vi "Create Data Folder.vi"(8 "error in (no error)":errorcluster, 9 "Description":string, 10 "Name":string, 11 "Parent Section":refnum<k24>) -> (0 "error out":errorcluster, 2 "New Section":refnum<k24>, 3 "Parent Section Duplicate":refnum<k24>, 4 "Newly Created?":bool)   [LabVIEW 2010, in "RefMem PtByPt System Definition API.lvlib"]
doc: "Creates a new folder for orginizational purposes."
uses:
  RefMem PtByPt System Definition API.lvlib
  NationalInstruments.VeriStand.SystemDefinitionAPI
  Custom Device/Controls/Global.vi
  Custom Device/RefMem PtByPt Custom Device.lvlib
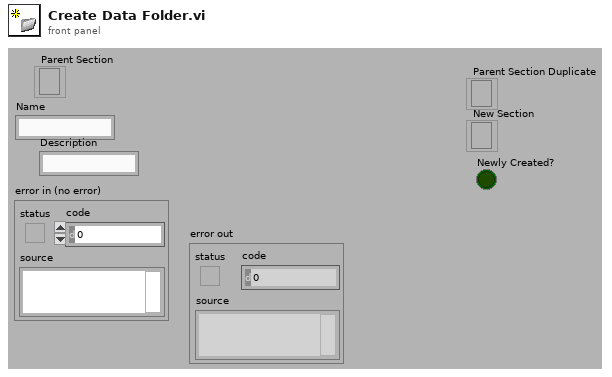
[diagram p1: front panel]
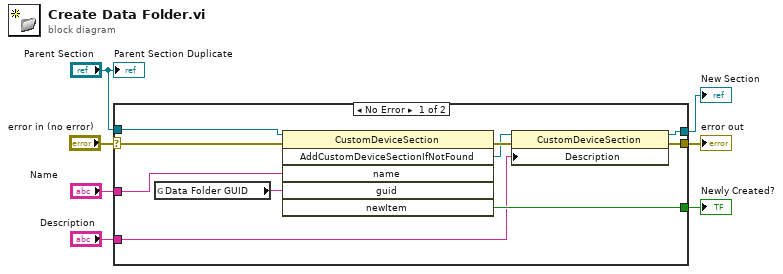
[diagram p0: block diagram]
diagram:
  n1 = case shown="No Error" "error in (no error)" {
    selector: "error in (no error)" -> [w16 w18]
    tunnel: [w10 w18] -> w7
    tunnel: "Parent Section" -> [w17 _]
    tunnel: "Name" -> [w15 _]
    tunnel: [w14 _] -> w5
    tunnel: "Description" -> [w11 _]
    tunnel: [w9 _] -> w1
    frame No Error {
      n2 = global read "Global.vi" "Data Folder GUID"() -> (w8:string)
      n3 = invoke class="CustomDeviceSection" method="AddCustomDeviceSectionIfNotFound"(reference=w17, error in=w16, "name"=w15, "guid"=w8) -> (error out=w13:errorcluster, "AddCustomDeviceSectionIfNotFound"=w12:refnum<k24>, "newItem"=w14:bool)  [unwired: 2 in, 3 out]
      n4 = property class="CustomDeviceSection"(reference=w12, error in=w13, "Description"=w11) -> (reference out=w9:refnum<k24>, error out=w10:errorcluster)
    }
    frame Error {
    }
  }
  "error out" <- w7
  "Newly Created?" <- w5
  "New Section" <- w1
  "Parent Section Duplicate" <- "Parent Section"
